vi "main.vi"() -> ()   [LabVIEW 2010]
uses:
  <vilib>/Native 3D Graph/xcontrol/3DPC_SurfacePlot.xctl
  PointCollection/x_y_z_enumeration.ctl
  PointCollection/PointCollection.lvclass
  PointCollection/mode_enum.ctl
panel:
  in  "buttonAddPoint":bool
  in  "point (x/y/z)":dbl[](array[numeric])
  in  "buttonFilter":bool
  out "result":dbl[][](array[numeric])
  in  "max (x/y/z)":dbl[](array[numeric])
  in  "min (x/y/z)":dbl[](array[numeric])
  in  "buttonSave":bool
  in  "increment step":dbl[unit]=0.017453292519943295
  out "rotation fit angles":dbl[unit][](array[numeric])
  out "scale factor":dbl
  out "translation vector (x/y/z)":dbl[](array[numeric])
  in  "buttonFit":bool
  in  "buttonRotate":bool
  in  "axis":T1
  in  "angle":dbl[unit]
  out "3D Graph":refnum<class "Base Datatype.lvclass">[](xcontrol)
  in  "buttonLoad":bool
  in  "buttonStop":bool
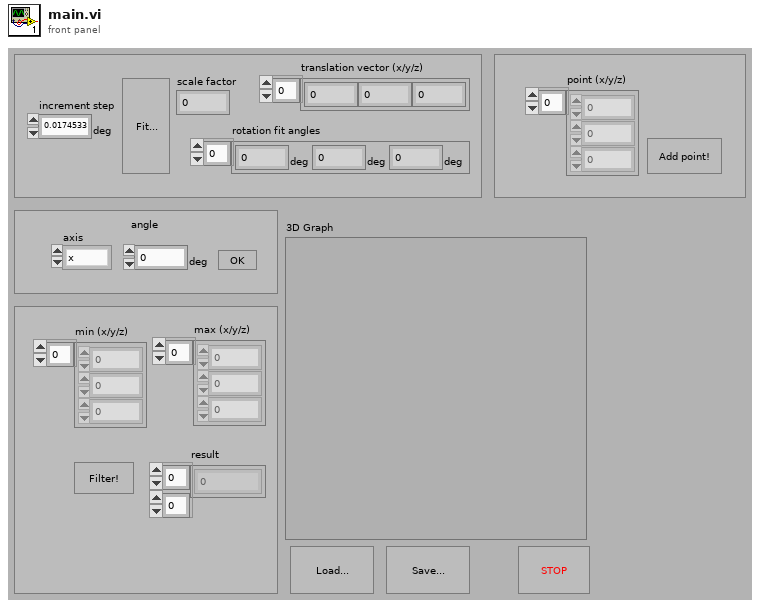
[diagram p1: front panel]
types:
  T1 = typedef "PointCollection.lvclass/x_y_z_enumeration.ctl" = enum16{"x", "y", "z"}
  T2 = typedef "PointCollection.lvclass/mode_enum.ctl" = enum16{"points first", "dimensions first"}
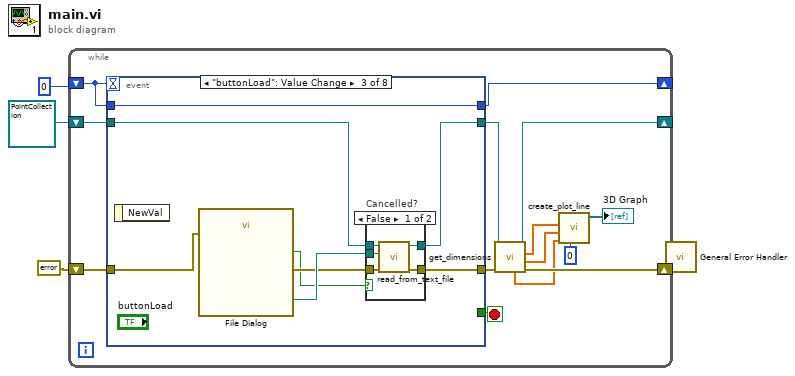
[diagram p0: block diagram]
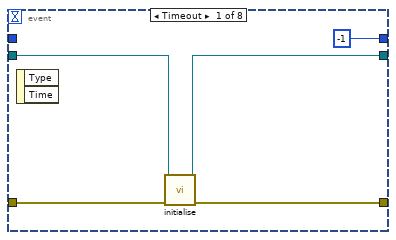
[diagram p2: hidden frame]
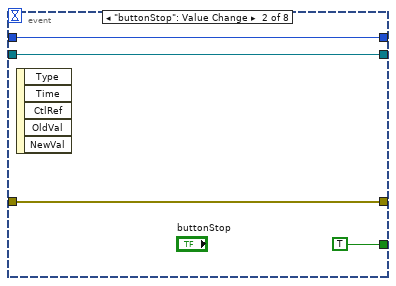
[diagram p3: hidden frame]
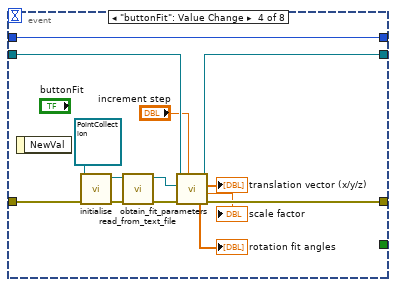
[diagram p5: hidden frame]
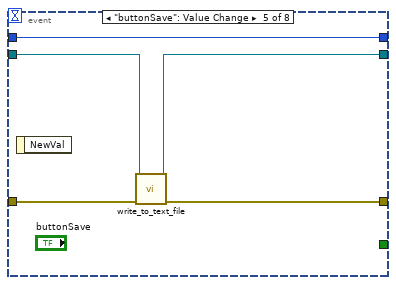
[diagram p6: hidden frame]
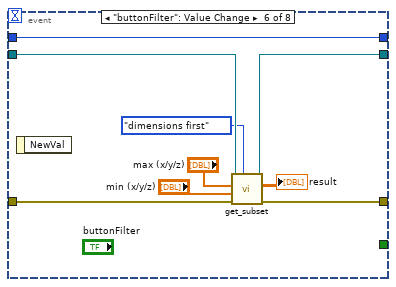
[diagram p7: hidden frame]
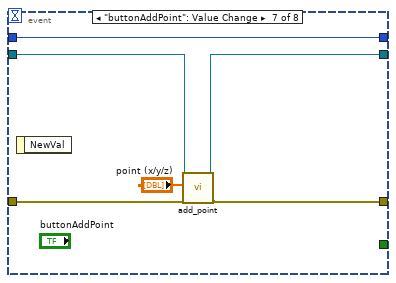
[diagram p8: hidden frame]
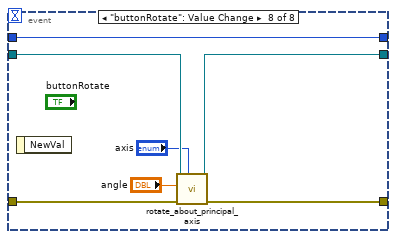
[diagram p9: hidden frame]
diagram:
  n1 = while {
    shift-right: [w17] -> _
    shift-left: 0 -> [w18]
    shift-right: [w8] -> w2
    shift-left: errorcluster {"status"=FALSE, "code"=0, "source"=""} ("error in (no error)") -> [w16]
    shift-right: [w12] -> _
    shift-left: refnum<class "PointCollection.lvclass"> refnum ("PointCollection.lvclass") -> [w14]
    stop <- w15 stop-if-true
    n2 = event shown="[2] \"buttonLoad\": Value Change" {
      selector: _ -> [_ _ _ _ _ _ _ _]
      dyn-events: _ -> [_ _ _ _ _ _ _ _]
      timeout: w18 -> [_ _ _ _ _ _ _ _]
      tunnel: [-1 w27 w35 w56 w61 w70 w76 w83] -> w17
      tunnel: w18 -> [_ w27 w35 w56 w61 w70 w76 w83]
      tunnel: [w19 w26 w34 w54 w59 w68 w74 w81] -> w13
      tunnel: w16 -> [w20 w26 w30 w47 w60 w69 w75 w82]
      tunnel: [_ TRUE _ _ _ _ _ _] -> w15
      tunnel: w14 -> [w22 w24 w32 w49 w58 w67 w72 w80]
      tunnel: [w21 w24 w31 w48 w57 w66 w71 w79] -> w11
      event Timeout {
        n3 = event-data() -> ()  [unwired: 1 in, 2 out]
        n4 = call "initialise.vi"("error in (no error)"=w20, "PointCollection in"=w22) -> ("error out"=w19:errorcluster, "PointCollection out"=w21:refnum<class "PointCollection.lvclass">)  [unwired: 8 in]
      }
      event "buttonStop": Value Change {
        n5 = event-data() -> ()  [unwired: 1 in, 5 out]
      }
      event "buttonLoad": Value Change {
        n6 = event-data() -> ()  [unwired: 1 in, 1 out]
        n7 = call "File Dialog"("error in"=w30) -> ("selected path"=w33:path, "cancelled"=w28:bool, "error out"=w29:errorcluster)  [unwired: 11 in, 1 out]
        n8 = case "Cancelled?" shown="False" w28 {
          tunnel: [w40 w42] -> w34
          tunnel: w33 -> [w39 _]
          tunnel: w32 -> [w38 w41]
          tunnel: [w37 w41] -> w31
          tunnel: w29 -> [w36 w42]
          frame False {
            n9 = call "read_from_text_file.vi"("error in (no error)"=w36, "file (use dialog)"=w39, "PointCollection in"=w38) -> ("error out"=w40:errorcluster, "PointCollection out"=w37:refnum<class "PointCollection.lvclass">)  [unwired: 7 in]
          }
          frame True {
          }
        }
      }
      event "buttonFit": Value Change {
        n10 = event-data() -> ()  [unwired: 1 in, 1 out]
        n11 = call "initialise.vi"("error in (no error)"=w47, "PointCollection in"=refnum<class "PointCollection.lvclass"> refnum ("PointCollection.lvclass")) -> ("error out"=w46:errorcluster, "PointCollection out"=w44:refnum<class "PointCollection.lvclass">)  [unwired: 8 in]
        n12 = call "read_from_text_file.vi"("error in (no error)"=w46, "PointCollection in"=w44) -> ("error out"=w55:errorcluster, "PointCollection out"=w53:refnum<class "PointCollection.lvclass">)  [unwired: 8 in]
        n13 = call-dynamic "obtain_fit_parameters.vi"("increment step"="increment step", "error in (no error)"=w55, "PointCollection B"=w53, "PointCollection in"=w49) -> ("error out"=w54:errorcluster, "scale factor"=→"scale factor":dbl, "translation vector"=→"translation vector (x/y/z)":dbl[], "PointCollection out"=w48:refnum<class "PointCollection.lvclass">, "rotation fit angles"=→"rotation fit angles":dbl[unit][])  [unwired: 3 in]
      }
      event "buttonSave": Value Change {
        n14 = event-data() -> ()  [unwired: 1 in, 1 out]
        n15 = call "write_to_text_file.vi"("error in (no error)"=w60, "PointCollection in"=w58) -> ("error out"=w59:errorcluster, "PointCollection out"=w57:refnum<class "PointCollection.lvclass">)  [unwired: 8 in]
      }
      event "buttonFilter": Value Change {
        n16 = event-data() -> ()  [unwired: 1 in, 1 out]
        n17 = call "get_subset.vi"("retrieval mode"=mode_enum."dimensions first", "error in (no error)"=w69, "min (x/y/z)"="min (x/y/z)", "max (x/y/z)"="max (x/y/z)", "PointCollection in"=w67) -> ("error out"=w68:errorcluster, "points"=→"result":dbl[][], "PointCollection out"=w66:refnum<class "PointCollection.lvclass">)  [unwired: 4 in]
      }
      event "buttonAddPoint": Value Change {
        n18 = event-data() -> ()  [unwired: 1 in, 1 out]
        n19 = call "add_point.vi"("error in (no error)"=w75, "point (x/y/z)"="point (x/y/z)", "PointCollection in"=w72) -> ("error out"=w74:errorcluster, "PointCollection out"=w71:refnum<class "PointCollection.lvclass">)  [unwired: 7 in]
      }
      event "buttonRotate": Value Change {
        n20 = event-data() -> ()  [unwired: 1 in, 1 out]
        n21 = call-dynamic "rotate_about_principal_axis.vi"("axis"="axis", "error in (no error)"=w82, "angle"="angle", "PointCollection in"=w80) -> ("error out"=w81:errorcluster, "PointCollection out"=w79:refnum<class "PointCollection.lvclass">)  [unwired: 6 in]
      }
    }
    n22 = call-dynamic "get_dimensions.vi"("error in (no error)"=w13, "PointCollection in"=w11) -> ("error out"=w8:errorcluster, "y"=w6:dbl[], "x"=w7:dbl[], "PointCollection out"=w12:refnum<class "PointCollection.lvclass">, "z"=w5:dbl[])  [unwired: 4 in, 1 out]
    n23 = call <vilib>:"create_plot_line.vi"("plot ID"=0 ("Plot ID"), "z vector"=w5, "y vector"=w6, "x vector"=w7) -> ("plots out"=→"3D Graph":refnum<class "Base Datatype.lvclass">[])  [unwired: 1 in, 6 out]
  }
  n24 = call <vilib>:"General Error Handler.vi"("error in (no error)"=w2) -> ()  [unwired: 10 in, 5 out]
